vi "CheckPanelEmpty.vi"(11 "Panel in":refnum<vi>) -> (2 "Empty?":bool)   [LabVIEW 2012, in "StimulCtrls.lvlib"]
uses:
  StimulCtrls.lvlib
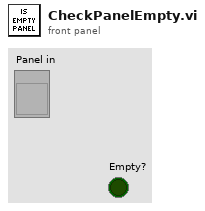
[diagram p1: front panel]
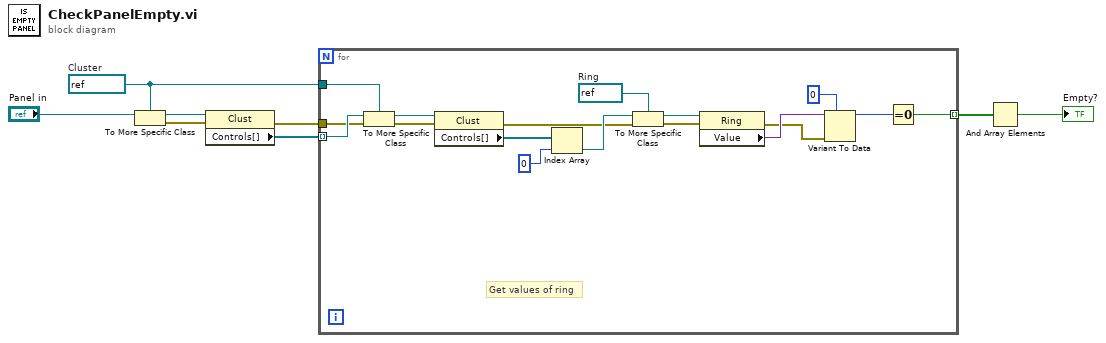
[diagram p0: block diagram]
diagram:
  w3 = refnum<vi> refnum  # Cluster
  n1 = To More Specific Class(target class=w3, reference="Panel in") -> (specific class reference=w7:refnum<vi>, error out=w6:errorcluster)  [unwired: 1 in]
  n2 = property class="Clust"(reference=w7, error in=w6) -> (error out=w4:errorcluster, "Controls[]"=w5:refnum<vi>[])  [unwired: 1 out]
  n3 = for {
    tunnel: w5 -> [w18] mode=indexing
    tunnel: w4 -> [w17]
    tunnel: w3 -> [w16]
    tunnel: [w9] -> w2 mode=indexing
    w24 = refnum<vi> refnum  # Ring
    # "Get values of ring"
    n4 = To More Specific Class(target class=w16, reference=w18, error in=w17) -> (specific class reference=w20:refnum<vi>, error out=w19:errorcluster)
    n5 = property class="Clust"(reference=w20, error in=w19) -> (error out=w14:errorcluster, "Controls[]"=w15:refnum<vi>[])  [unwired: 1 out]
    n6 = Index Array(array=w15, index=0) -> (element=w23:refnum<vi>)
    n7 = To More Specific Class(target class=w24, reference=w23, error in=w14) -> (specific class reference=w22:refnum<vi>, error out=w21:errorcluster)
    n8 = property class="Ring"(reference=w22, error in=w21) -> (error out=w12:errorcluster, "Value"=w13:variant)  [unwired: 1 out]
    n9 = Variant To Data(error in=w12, type=0, Variant=w13) -> (data=w10:i32)  [unwired: 1 out]
    n10 = Equal To 0?(x=w10) -> (x = 0?=w9:bool)
  }
  n11 = And Array Elements(Boolean array=w2) -> (logical AND=→"Empty?":bool)
